vi "Ramp EG&G 5210 DAC.vi"(0 "GPIB Address":refnum<visa-resource-name>) -> ()   [LabVIEW 2020]
panel:
  in  "Starting Set Point":dbl format="%.3f"
  out "?":i32
  out "?":i32
  out "?":i32
  in  "Set Point":dbl format="%.3f"
  in  "STOP":bool
  in  "Rate V/S":dbl=0.1 format="%.2f"
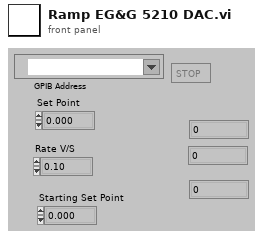
[diagram p1: front panel]
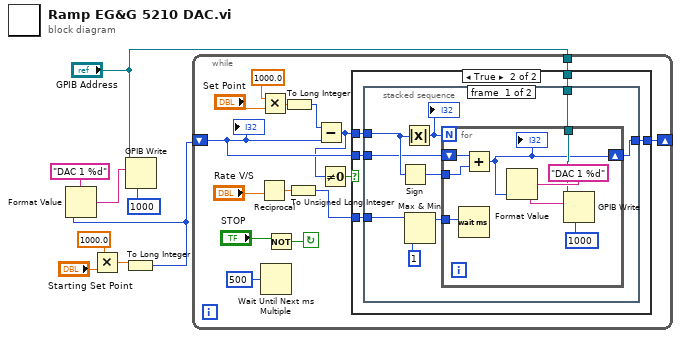
[diagram p0: block diagram]
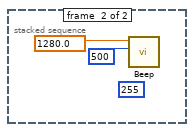
[diagram p3: hidden frame]
diagram:
  n1 = Multiply(x=1000.0, y="Starting Set Point") -> (x*y=w5:dbl)
  n2 = To Long Integer(number=w5) -> (32bit integer=w2:i32)
  n3 = Format Value(format string="DAC 1 %d", value (0)=w2) -> (output string=w3:string)  [unwired: 1 in]
  n4 = GPIB Write(0:"GPIB Address", 1:w3, 4:1000) -> ()  [unwired: 2 in, 2 out]
  n5 = while {
    tunnel: "GPIB Address" -> [w15]
    shift-left: w2 -> [w13]
    shift-right: [w14] -> _
    stop <- w18 continue-if-true
    n6 = Reciprocal(x="Rate V/S") -> (1/x=w16:dbl)
    n7 = Multiply(x=1000.0, y="Set Point") -> (x*y=w20:dbl)
    n8 = Wait Until Next ms Multiple(millisecond multiple=u32 500) -> ()  [unwired: 1 out]
    n9 = Not(x="STOP") -> (.not. x?=w18:bool)
    n10 = To Long Integer(number=w20) -> (32bit integer=w17:i32)
    n11 = To Unsigned Long Integer(number=w16) -> (unsigned 32bit integer=w12:u32)
    n12 = Subtract(x=w17, y=w13) -> (x-y=w11:i32)
    n13 = Not Equal To 0?(x=w11) -> (x != 0?=w10:bool)
    n14 = case shown="True" w10 {
      tunnel: w12 -> [_ w25]
      tunnel: w13 -> [w24 w26]
      tunnel: w11 -> [_ w27]
      tunnel: [w24 w28] -> w14
      tunnel: w15 -> [_ w29]
      frame False {
      }
      frame True {
        n15 = stacked-sequence {
          tunnel: w25 -> [w30 _]
          tunnel: w26 -> [w31 _]
          tunnel: w27 -> [w32 _]
          tunnel: [w33 _] -> w28
          tunnel: w29 -> [w34 _]
          frame #0 {
            n16 = Sign(1:w32) -> (0:w35:i32)
            n17 = Absolute Value(x=w32) -> (abs(x)=w36:i32)
            "?" <- w36
            n18 = Max & Min(x=w30, y=1) -> (max(x,y)=w37:u32)  [unwired: 1 out]
            n19 = for {
              N: w36 -> [_]
              shift-right: [w40] -> w33
              shift-left: w31 -> [w41]
              tunnel: w37 -> [w39]
              tunnel: w35 -> [w42]
              tunnel: w34 -> [w43]
              n20 = Wait (ms)(milliseconds to wait=w39) -> ()  [unwired: 1 out]
              n21 = Add(x=w41, y=w42) -> (x+y=w40:i32)
              "?" <- w40
              n22 = Format Value(format string="DAC 1 %d", value (0)=w40) -> (output string=w44:string)  [unwired: 1 in]
              n23 = GPIB Write(0:w43, 1:w44, 4:u32 1000) -> ()  [unwired: 2 in, 2 out]
            }
          }
          frame #1 {
            (unwired) i16 255
            n24 = call <vilib>:"Beep.vi"("duration (msec) - ignored"=i16 500, "frequency (Hz) - ignored"=1280.0) -> ()  [unwired: 10 in]
          }
        }
      }
    }
    "?" <- w13
  }
